vi "Write TsQue.vi"(8 "error in (no error)":errorcluster, 10 "TsQue":refnum<queue>, 11 "NiDaqMx in":refnum<class "NiDaqMx.lvclass">) -> (0 "error out":errorcluster, 3 "NiDaqMx out":refnum<class "NiDaqMx.lvclass">)   [LabVIEW 2018, in "DigitizerPlugins.lvlib" / "NiDaqMx.lvclass"]
uses:
  NiDaqMx.lvclass
  NiDaqMx.lvclass/NiDaqMx.ctl
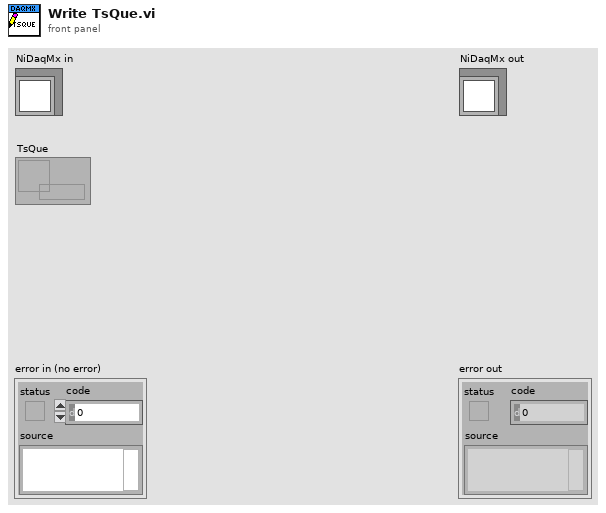
[diagram p1: front panel]
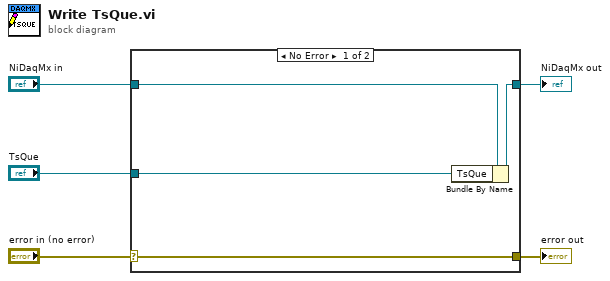
[diagram p0: block diagram]
diagram:
  n1 = case shown="No Error" "error in (no error)" {
    selector: "error in (no error)" -> [w9 w10]
    tunnel: [w9 w10] -> w4
    tunnel: [w7 w11] -> w2
    tunnel: "NiDaqMx in" -> [w8 w11]
    tunnel: "TsQue" -> [w6 _]
    frame No Error {
      n2 = Bundle By Name(cluster=w8, "TsQue"=w6) -> (w7:refnum<class "NiDaqMx.lvclass">)
    }
    frame Error {
    }
  }
  "error out" <- w4
  "NiDaqMx out" <- w2
